vi "From CSV File.vi"(8 "error in (no error)":errorcluster, 9 "Path":path, 10 "engine in":refnum<class "engine configuration.lvclass">, 11 "Add Module editor node in":refnum<class "Add Module editor node.lvclass">) -> (0 "error out":errorcluster, 1 "Update":bool, 2 "engine out":refnum<class "engine configuration.lvclass">, 3 "Add Module editor node out":refnum<class "Add Module editor node.lvclass">)   [LabVIEW 2018, in "Add Module editor node.lvclass"]
uses:
  Add Module editor node.lvclass
  <vilib>/NI/Module Execution Interface/Engine Configuration/engine configuration.lvclass
  module/configuration/Add Module configuration.lvclass
  C:/Program Files (x86)/National Instruments/LabVIEW 2018/vi.lib/NI/Configuration Framework/serializable configuration/NISE_CEF_serializable configuration.lvclass
  <vilib>/NI/Configuration Framework/serializable configuration/NISE_CEF_serializable configuration.lvclass/NISE_CEF_serializable configuration.ctl
  module/configuration/Add Module configuration.lvclass/Add Module configuration.ctl
  <vilib>/Utility/LVClass/Get LV Class Name.vi
  <vilib>/NI/Configuration Framework/error generator/NISE_error generator.vi
  <vilib>/NI/Tag Bus Module Framework/channel/TBM channel.lvclass
  <vilib>/NI/Configuration Framework/serializable configuration/NISE_CEF_serializable configuration.lvclass
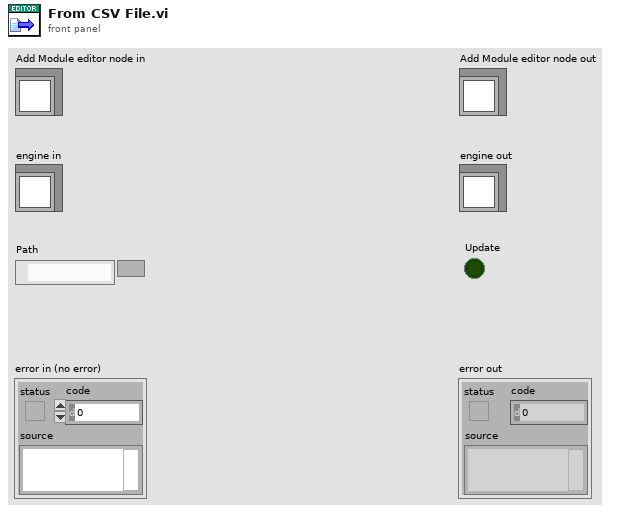
[diagram p1: front panel]
types:
  T1 = typedef "Add Module configuration.lvclass/Line.ctl" = cluster{"channel":refnum<class "TBM channel.lvclass">}
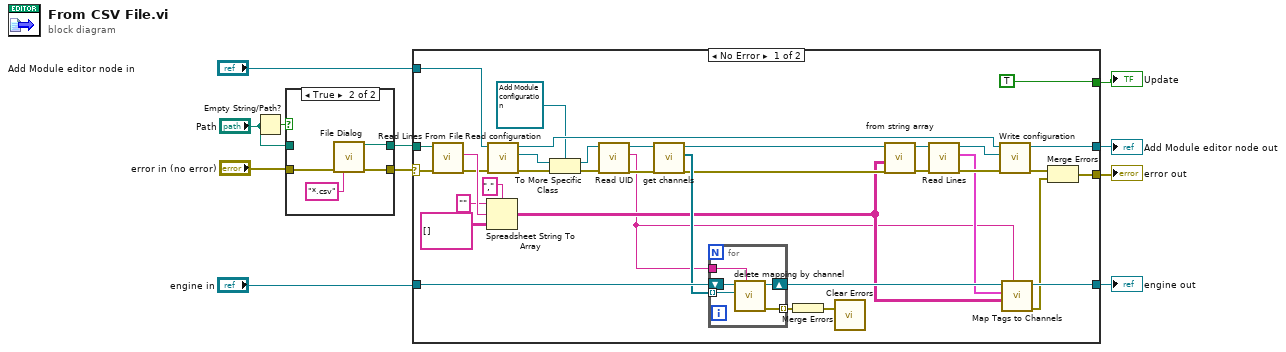
[diagram p0: block diagram]
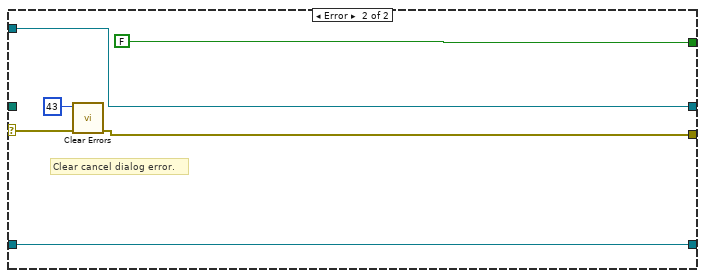
[diagram p2: hidden frame]
diagram:
  n1 = Empty String/Path?(string/path="Path") -> (empty?=w11:bool)
  n2 = case shown="True" w11 {
    tunnel: "error in (no error)" -> [w12 w16]
    tunnel: [w12 w15] -> w7
    tunnel: [w13 w14] -> w8
    tunnel: "Path" -> [w13 _]
    frame False {
    }
    frame True {
      n3 = call "File Dialog"("error in"=w16, "pattern (all files)"="*.csv") -> ("selected path"=w14:path, "error out"=w15:errorcluster)  [unwired: 10 in, 2 out]
    }
  }
  n4 = case shown="No Error" w7 {
    selector: w7 -> [w46 w61]
    tunnel: [w36 w60] -> w1
    tunnel: [w30 w63] -> w3
    tunnel: "Add Module editor node in" -> [w35 w63]
    tunnel: w8 -> [w51 _]
    tunnel: [TRUE ("Update") FALSE ("Update")] -> w4
    tunnel: "engine in" -> [w43 w58]
    tunnel: [w37 w58] -> w2
    frame No Error {
      n5 = call <vilib>:"Read Lines From File.vi"("file path (dialog if empty)"=w51, "error in (not an error)"=w46) -> ("line string"=w49:string, "error out"=w34:errorcluster)  [unwired: 5 in, 1 out]
      n6 = Spreadsheet String To Array(delimiter (Tab)=",", format string="", spreadsheet string=w49, array type (2D Dbl)=string[][] [] ("type (empty)")) -> (array=w19:string[][])
      n7 = call-dynamic "Read configuration.vi"("error in"=w34, "Add Module editor node in"=w35) -> ("error out"=w32:errorcluster, "configuration"=w33:refnum<class "NISE_CEF_serializable configuration.lvclass">, "Add Module editor node out"=w31:refnum<class "Add Module editor node.lvclass">)  [unwired: 7 in]
      n8 = To More Specific Class(target class=refnum<class "Add Module configuration.lvclass"> refnum ("tag bus configurable plugin module configuration"), reference=w33, error in=w32) -> (specific class reference=w45:refnum<class "Add Module configuration.lvclass">, error out=w39:errorcluster)
      n9 = call <vilib>:"Read UID.vi"("error in"=w39, "configuration in"=w45) -> ("error out"=w27:errorcluster, "instance id"=w18:string, "configuration out"=w44:refnum<class "Add Module configuration.lvclass">)  [unwired: 7 in]
      n10 = call-dynamic "get channels.vi"("Add Module configuration in"=w44) -> ("channels"=w42:refnum<class "TBM channel.lvclass">[], "Add Module configuration out"=w40:refnum<class "Add Module configuration.lvclass">)  [unwired: 9 in]
      n11 = for {
        tunnel: w18 -> [w56]
        tunnel: w42 -> [w55] mode=indexing
        tunnel: [w54] -> w41 mode=indexing
        shift-right: [w53] -> w38
        shift-left: w43 -> [w57]
        n12 = call <vilib>:"delete mapping by channel.vi"("owner ID"=w56, "channel"=w55, "engine configuration in"=w57) -> ("error out"=w54:errorcluster, "engine configuration out"=w53:refnum<class "engine configuration.lvclass">)  [unwired: 7 in]
      }
      n13 = Merge Errors(w41) -> (w28:errorcluster)
      n14 = call <vilib>:"Clear Errors.vi"("error in (no error)"=w28) -> ()  [unwired: 5 in, 2 out]
      n15 = call-dynamic "from string array.vi"("error in (no error)"=w27, "String Array"=w19, "Add Module configuration in"=w40) -> ("error out"=w25:errorcluster, "Add Module configuration out"=w22:refnum<class "Add Module configuration.lvclass">)  [unwired: 7 in]
      n16 = call "Read Lines.vi"("error in (no error)"=w25, "Add Module configuration in"=w22) -> ("error out"=w24:errorcluster, "Lines"=w20:T1[], "Add Module configuration out"=w23:refnum<class "Add Module configuration.lvclass">)  [unwired: 7 in]
      n17 = call-dynamic "Write configuration.vi"("error in"=w24, "configuration"=w23, "Add Module editor node in"=w31) -> ("error out"=w29:errorcluster, "Add Module editor node out"=w30:refnum<class "Add Module editor node.lvclass">)  [unwired: 7 in]
      n18 = call "Map Tags to Channels.vi"("instance id"=w18, "String Array"=w19, "Lines"=w20, "engine configuration in"=w38) -> ("error out"=w21:errorcluster, "engine configuration out"=w37:refnum<class "engine configuration.lvclass">)  [unwired: 6 in]
      n19 = Merge Errors(w29, w21) -> (w36:errorcluster)
    }
    frame Error {
      # "Clear cancel dialog error."
      n20 = call <vilib>:"Clear Errors.vi"("error in (no error)"=w61, "specific error code to clear (0: all)"=43) -> ("error out"=w60:errorcluster)  [unwired: 4 in, 1 out]
    }
  }
  "error out" <- w1
  "Add Module editor node out" <- w3
  "Update" <- w4
  "engine out" <- w2
